vi "MI.Get DBL.vi"(8 "error in (no error)":errorcluster, 10 "String":string, 11 "TCP Network Connection in":refnum<k5>) -> (0 "error out":errorcluster, 2 "Numeric":dbl, 3 "TCP Network Connection out":refnum<k5>)   [LabVIEW 2016, in "instrument.Cryostation.lvclass"]
uses:
  instrument.Cryostation.lvclass
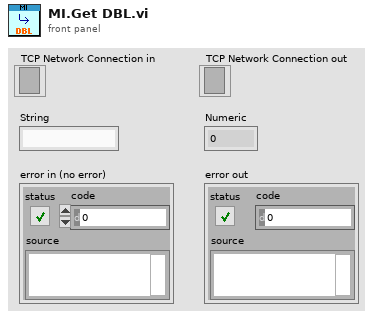
[diagram p1: front panel]
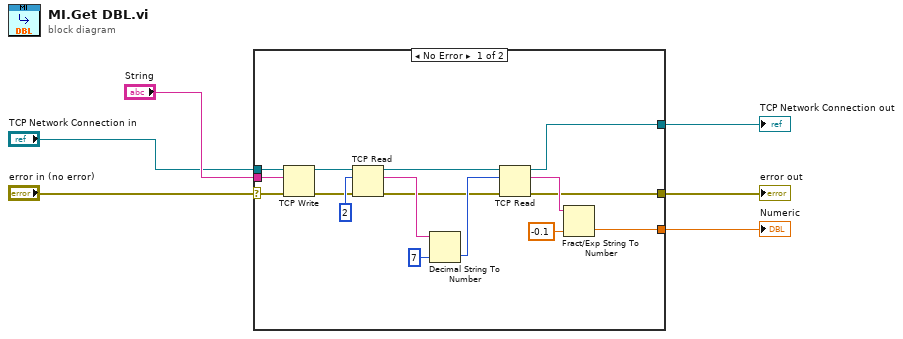
[diagram p0: block diagram]
diagram:
  n1 = case shown="No Error" "error in (no error)" {
    selector: "error in (no error)" -> [w7 w24]
    tunnel: [w22 w23] -> w6
    tunnel: "String" -> [w21 _]
    tunnel: "TCP Network Connection in" -> [w10 w23]
    tunnel: [w9 _] -> w3
    tunnel: [w8 w24] -> w2
    frame No Error {
      n2 = TCP Write(connection ID=w10, data in=w21, error in (no error)=w7) -> (connection ID out=w19:refnum<k5>, error out=w18:errorcluster)  [unwired: 1 in, 1 out]
      n3 = TCP Read(connection ID=w19, bytes to read=2, error in (no error)=w18) -> (connection ID out=w14:refnum<k5>, data out=w17:string, error out=w13:errorcluster)  [unwired: 2 in]
      n4 = Decimal String To Number(string=w17, default (0L)=7 ("default (0 I32)")) -> (number=w15:i32)  [unwired: 1 in, 1 out]
      n5 = TCP Read(connection ID=w14, bytes to read=w15, error in (no error)=w13) -> (connection ID out=w22:refnum<k5>, data out=w12:string, error out=w8:errorcluster)  [unwired: 2 in]
      n6 = Fract/Exp String To Number(string=w12, default (0 dbl)=-0.1 ("default (0 DBL)")) -> (number=w9:dbl)  [unwired: 2 in, 1 out]
    }
    frame Error {
    }
  }
  "TCP Network Connection out" <- w6
  "Numeric" <- w3
  "error out" <- w2
